vi "Insert_Into_Array_1D_Element.vi"(9 "Element IIA":i8, 10 "Index IIA":i32, 11 "Insert Into Array 1D":i8[](array[numeric])=[1, 2, 3, 4]) -> (3 "Array 1D IIA":i8[](array[numeric])=[1, 2, 3, 4])   [LabVIEW 2018]
panel:
  out "Iteration":i32
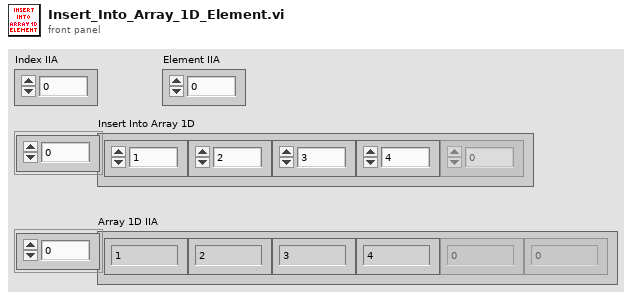
[diagram p1: front panel]
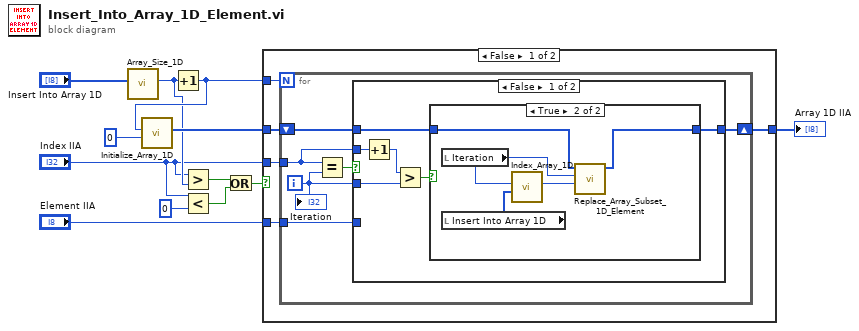
[diagram p0: block diagram]
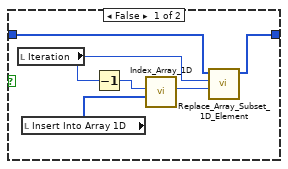
[diagram p2: hidden frame]
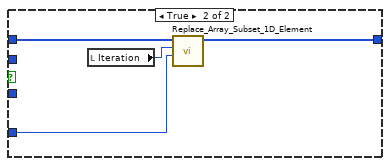
[diagram p3: hidden frame]
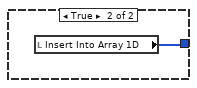
[diagram p4: hidden frame]
diagram:
  n1 = call "Array_Size_1D.vi"("Array"="Insert Into Array 1D") -> ("Size"=w6:i32)  [unwired: 10 in]
  n2 = Increment(x=w6) -> (x+1=w7:i32)
  n3 = call "Initialize_Array_1D.vi"("Value"=i8 0, "Dimension 1D Array"=w7) -> ("Initialized Array 1D"=w12:i8[])  [unwired: 9 in]
  n4 = Greater?(x="Index IIA", y=w6) -> (0:w4:bool)
  n5 = Less?(x="Index IIA", y=0) -> (x < y?=w3:bool)
  n6 = Or(x=w4, y=w3) -> (x .or. y?=w5:bool)
  n7 = case shown="False" w5 {
    tunnel: w12 -> [w17 _]
    tunnel: w7 -> [w16 _]
    tunnel: [w15 w45] -> w10
    tunnel: "Index IIA" -> [w14 _]
    tunnel: "Element IIA" -> [w13 _]
    frame False {
      n8 = for {
        N: w16 -> [_]
        tunnel: w14 -> [w18]
        tunnel: w13 -> [w20]
        shift-right: [w21] -> w15
        shift-left: w17 -> [w22]
        i -> [w19]
        n9 = Equal?(x=w18, y=w19) -> (x = y?=w23:bool)
        n10 = case shown="False" w23 {
          tunnel: w22 -> [w25 w44]
          tunnel: [w24 w43] -> w21
          tunnel: w20 -> [_ w41]
          tunnel: w19 -> [w27 _]
          tunnel: w18 -> [w26 _]
          frame False {
            n11 = Increment(x=w26) -> (x+1=w28:i32)
            n12 = Greater?(x=w28, y=w27) -> (0:w29:bool)
            n13 = case shown="True" w29 {
              tunnel: w25 -> [w34 w39]
              tunnel: [w33 w36] -> w24
              frame False {
                n14 = local read "Iteration"() -> (w30:i32)
                n15 = local read "Insert Into Array 1D"() -> (w32:i8[])
                n16 = Decrement(x=w30) -> (x-1=w31:i32)
                n17 = call "Index_Array_1D.vi"("Index Array 1D"=w32, "Index"=w31) -> ("Value"=w35:i8)  [unwired: 9 in]
                n18 = call "Replace_Array_Subset_1D_Element.vi"("Element RAS"=w35, "Index RAS1D"=w30, "RAS1D"=w34) -> ("New Array RAS1D"=w33:i8[])  [unwired: 8 in]
              }
              frame True {
                n19 = local read "Iteration"() -> (w38:i32)
                n20 = local read "Insert Into Array 1D"() -> (w40:i8[])
                n21 = call "Index_Array_1D.vi"("Index Array 1D"=w40, "Index"=w38) -> ("Value"=w37:i8)  [unwired: 9 in]
                n22 = call "Replace_Array_Subset_1D_Element.vi"("Element RAS"=w37, "Index RAS1D"=w38, "RAS1D"=w39) -> ("New Array RAS1D"=w36:i8[])  [unwired: 8 in]
              }
            }
          }
          frame True {
            n23 = local read "Iteration"() -> (w42:i32)
            n24 = call "Replace_Array_Subset_1D_Element.vi"("Element RAS"=w41, "Index RAS1D"=w42, "RAS1D"=w44) -> ("New Array RAS1D"=w43:i8[])  [unwired: 8 in]
          }
        }
        "Iteration" <- w19
      }
    }
    frame True {
      n25 = local read "Insert Into Array 1D"() -> (w45:i8[])
    }
  }
  "Array 1D IIA" <- w10
